vi "Read MP Registry Data.vi"(7 "Micropulse # In":i32, 8 "error in (no error)":errorcluster) -> (0 "error out":errorcluster, 2 "Micropulse Data":T2={"Instrument Type"=enum."MicroPulse 5", "Serial #"=0, "Sample Frequency"=enum."100MHz", "dt (us)"=0.0, "DOF"=enum."8-bit Mode", "Material Velocity"=1.0, "Asynch Reads"=enum."Disabled", "NUM of Tests"=0, "System Details"={"System Type"=enum."MicroPulse 5", "Serial No."=0, "Channels"={"Conv"=0, "PA"=0, "Extra"=0}, "Sample Frequency"={"Default"=0, "Actual"=0}, "Software Versions"="", "Data Output Format"={"Default"=enum."8-bit Mode", "Actual"=enum."8-bit Mode"}, "Temperatures"={"System"=0, "Processor"=0, "Slave Sys"=0, "Slave Proc"=0}, "Tx Buffer Size"=0, "System Error"="", "No. of Cards"=0, "DAC Gain"=0, "Uptimes"={"since Power"=0, "since RSTS"=0, "since SRST"=0}, "Voltages"=[], "Interface Cards"=[]}, "Gates"=[], "Encoders"=[], "CMD LUT"=variant, "Command List"=""} {"System Details"."Interface Cards"."FPGA - T" format="%.0f °C"; "System Details"."Interface Cards"."Board - T" format="%.0f °C"; "System Details"."Voltages"."Difference" format="%.2fV"; "System Details"."Voltages"."Measured" format="%.2fV"; "System Details"."Voltages"."Nominal" format="%.2fV"; "System Details"."DAC Gain" format="%.0fdB"; "System Details"."Tx Buffer Size" format="%.0fMB"; "System Details"."Temperatures"."Slave Proc" format="%.0f C"; "System Details"."Temperatures"."Slave Sys" format="%.0f C"; "System Details"."Temperatures"."Processor" format="%.0f C"; "System Details"."Temperatures"."System" format="%.0f C"; "System Details"."Sample Frequency"."Actual" format="%.0fMHz"; "System Details"."Sample Frequency"."Default" format="%.0fMHz"; "Encoders"."Encoder Filter" max=255; "Encoders"."Backlash Period (s)" min=0.0005 max=10.0 step=0.0005; "Encoders"."Multiplier" min=1 max=100000; "Encoders"."Counts/mm" min=1 max=100000; "Gates"."Insp Gates"."Max # Peaks" max=64000 step=100; "Gates"."Insp Gates"."Threshold" min=10 max=4095 step=10; "Gates"."Insp Gates"."Length (us)" min=0.0 max=96000.0 step=100.0; "Gates"."Insp Gates"."Start (us)" min=0.0 max=64000.0 step=100.0; "Gates"."Echo Gate"."Threshold" min=10 max=4095 step=10; "Gates"."Echo Gate"."Length (us)" min=0.0 max=96000.0 step=100.0; "Gates"."Echo Gate"."Start (us)" min=0.0 max=64000.0 step=100.0; "Gates"."Display Gate"."Length" min=0.0 max=64000.0 step=1000.0; "Gates"."Display Gate"."Start" min=0.0 max=64000.0 step=1000.0}, 3 "TCP config":T1={"Connection ID"=refnum, "IP address"="10.1.1.2", "host port"=1067, "OC timeout"=-1, "Read timeout"=0, "Write timeout"=0} {"Write timeout" format="%dms"; "Read timeout" format="%dms"; "OC timeout" format="%dms"}, 5 "Micropulse # Out":i32)   [LabVIEW 2026, in "MicroPulse_Driver.lvlib"]
doc: "The specified test(s) is repeated until a new mode (for example: STL or STX) is requested. The data is buffered for each cycle, i.e. if a single test is requested then data is output between each test, if all tests requested then data for each cycle of tests is buffered and output. The tests within a cycle are fired at the requested PRF (subject to gates set not being longer than the PRF). The next cycle will not start until this data has been output.\nParameters:\n<Tn> : Test number. An integer value from 0 to the maximum number of tests (default maximum is 1279 tests).\nTn = 0 for all conventional tests. If the S extension is used it applies to all tests in the sweep number specified: 1-32, 0 = all sweeps\n\nExample:\nNUM 100\nSTP 0 : MicroPulse sends data for tests 1 to 100 repeatedly\nSTL 1 : After completing the reporting of the data from the last test cycle, the MicroPulse enters STL mode on test 1."
uses:
  MicroPulse_Driver.lvlib
  Datatypes/MP-Registry Data-Cluster.ctl
  <instrlib>/MicroPulse/Public/Data/Datatypes/MP - instrument type.ctl
  Datatypes/MP - sample frequency.ctl
  Datatypes/MP - data output format.ctl
  Datatypes/MP - asynch read mode.ctl
  Datatypes/MP - general system status.ctl
  Datatypes/MP - interface card status.ctl
  Datatypes/subdatatypes/MP - Registry Gates.ctl
  Datatypes/MP - display gate.ctl
  Datatypes/MP - echo gate mode.ctl
  Datatypes/MP - echo gate parameters.ctl
  Datatypes/MP - multigate inspection gate parameters.ctl
  Datatypes/MP - hysteresis level.ctl
  Datatypes/MP - multigate mode.ctl
  Datatypes/MP - encoder settings.ctl
  Datatypes/MP - encoder type.ctl
  Datatypes/TCP config.ctl
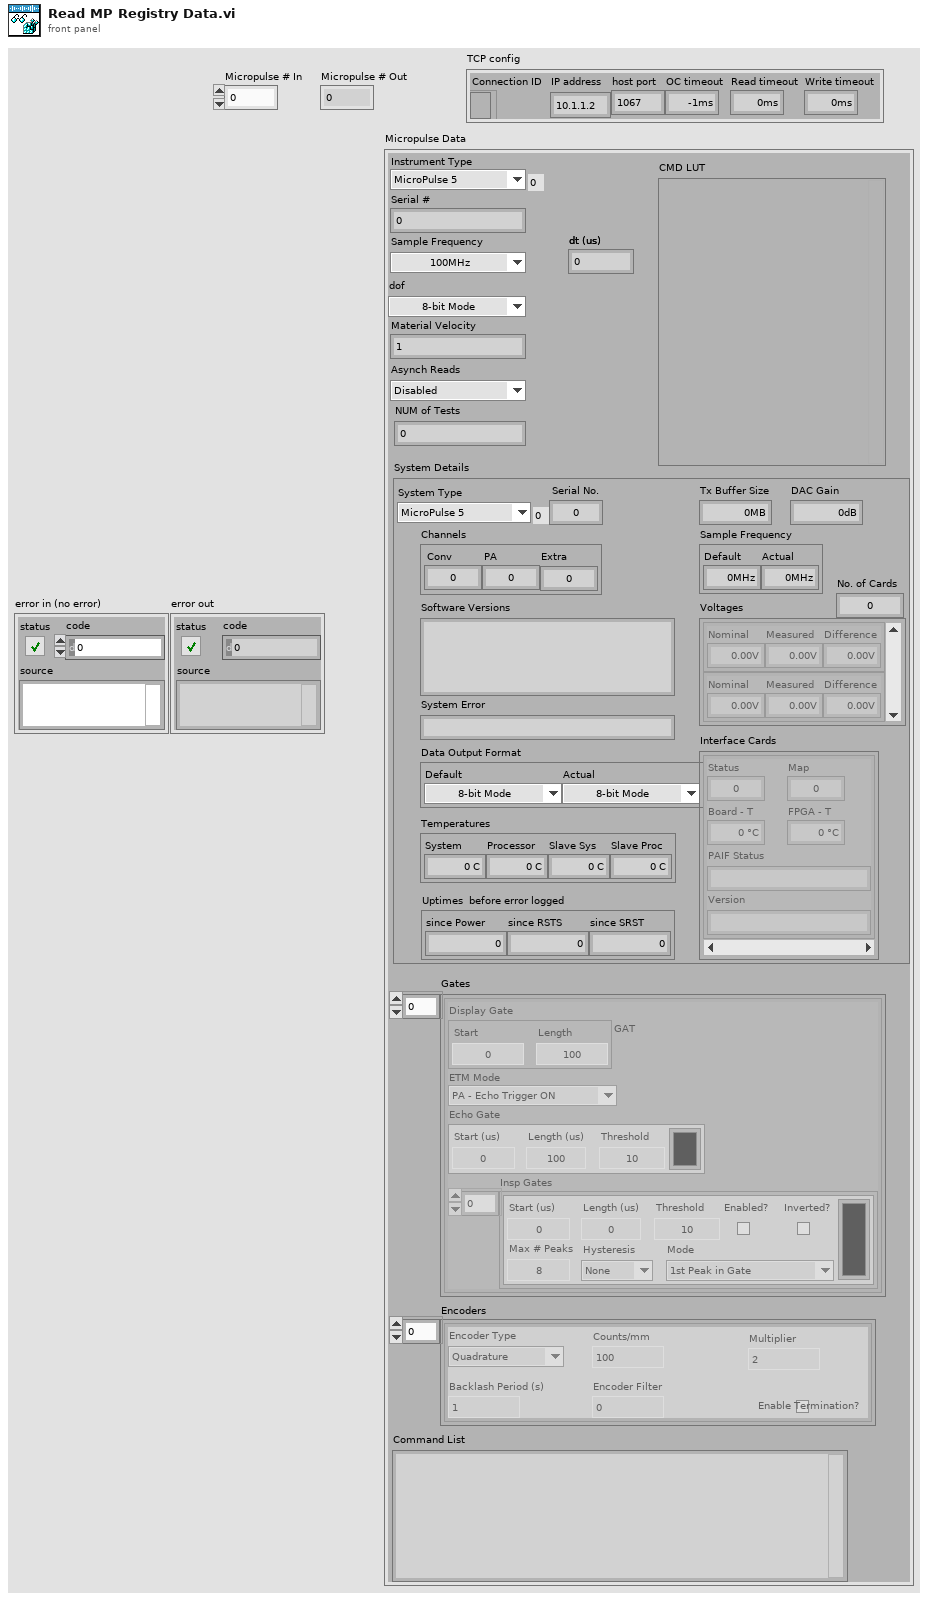
[diagram p1: front panel]
types:
  T1 = typedef "MicroPulse_Driver.lvlib/TCP config.ctl" = cluster{"Connection ID":refnum<k5>, "IP address":string, "host port":u16, "OC timeout":i32, "Read timeout":i32, "Write timeout":i32}
  T2 = typedef "MicroPulse_Driver.lvlib/MP-Registry Data-Cluster.ctl" = cluster{"Instrument Type":T3, "Serial #":u64, "Sample Frequency":T4, "dt (us)":dbl, "DOF":T5, "Material Velocity":dbl, "Asynch Reads":T6, "NUM of Tests":u32, "System Details":T7, "Gates":T9[], "Encoders":T16[], "CMD LUT":variant, "Command List":string}
  T3 = typedef "MicroPulse_Driver.lvlib/MP - instrument type.ctl" = enum16{"MicroPulse 5", "LT1", "LT2", "LTPA", "MPLT", "MicroPulse 6", "PipeScanner", "<MicroPulse>", "Micropulse 4", "Simulated Data"}
  T4 = typedef "MicroPulse_Driver.lvlib/MP - sample frequency.ctl" = enum16{"Use Default", "200MHz (LT2 only)", "100MHz", "50MHz", "25MHz", "10MHz"}
  T5 = typedef "MicroPulse_Driver.lvlib/MP - data output format.ctl" = enum16{"", "8-bit Mode", "10-bit Mode", "12-bit Mode", "16-bit Mode", "8-bit Log Mode", "12-bit Packed Mode"}
  T6 = typedef "MicroPulse_Driver.lvlib/MP - asynch read mode.ctl" = enum16{"Disabled", "Enabled"}
  T7 = typedef "MicroPulse_Driver.lvlib/MP - general system status.ctl" = cluster{"System Type":T3, "Serial No.":u64, "Channels":cluster{"Conv":u8, "PA":u16, "Extra":u32}, "Sample Frequency":cluster{"Default":u8, "Actual":u8}, "Software Versions":string, "Data Output Format":cluster{"Default":T5, "Actual":T5}, "Temperatures":cluster{"System":u8, "Processor":u8, "Slave Sys":u8, "Slave Proc":u8}, "Tx Buffer Size":u32, "System Error":string, "No. of Cards":u8, "DAC Gain":i16, "Uptimes":cluster{"since Power":u32, "since RSTS":u32, "since SRST":u32}, "Voltages":cluster{"Nominal":dbl, "Measured":dbl, "Difference":dbl}[], "Interface Cards":T8[]}
  T8 = typedef "MicroPulse_Driver.lvlib/MP - interface card status.ctl" = cluster{"Status":u8, "Map":u8, "Board - T":u8, "FPGA - T":u8, "PAIF Status":string, "Version":string}
  T9 = typedef "MicroPulse_Driver.lvlib/MP - Registry Gates.ctl" = cluster{"Display Gate":T10, "ETM Mode":T11, "Echo Gate":T12, "Insp Gates":T13[]}
  T10 = typedef "MicroPulse_Driver.lvlib/MP - display gate.ctl" = cluster{"Start":dbl, "Length":dbl}
  T11 = typedef "MicroPulse_Driver.lvlib/MP - echo gate mode.ctl" = enum16{"Echo Trigger OFF", "Echo Gate Display Mode", "Echo Trigger ON", "Multi Gate or FMC Mode", "Reserved", "PA - Echo Trigger ON"}
  T12 = typedef "MicroPulse_Driver.lvlib/MP - echo gate parameters.ctl" = cluster{"Start (us)":dbl, "Length (us)":dbl, "Threshold":u16, "Colour":u32}
  T13 = typedef "MicroPulse_Driver.lvlib/MP - multigate inspection gate parameters.ctl" = cluster{"Start (us)":dbl, "Length (us)":dbl, "Threshold":u16, "Enabled?":bool, "Max # Peaks":u16, "Hysteresis":T14, "Mode":T15, "Inverted?":bool, "Colour ":u32}
  T14 = typedef "MicroPulse_Driver.lvlib/MP - hysteresis level.ctl" = enum16{"None", "3dB", "6dB", "9dB", "12dB"}
  T15 = typedef "MicroPulse_Driver.lvlib/MP - multigate mode.ctl" = enum16{"1st Peak in Gate", "Largest Peak In Gate", "All Peaks In Gate", "1st Threshold Crossing"}
  T16 = typedef "MicroPulse_Driver.lvlib/MP - encoder settings.ctl" = cluster{"Encoder Type":T17, "Counts/mm":u32, "Enable Termination?":bool, "Multiplier":u32, "Backlash Period (s)":dbl, "Encoder Filter":u32}
  T17 = typedef "MicroPulse_Driver.lvlib/MP - encoder type.ctl" = enum16{"Quadrature", "Step/Direction"}
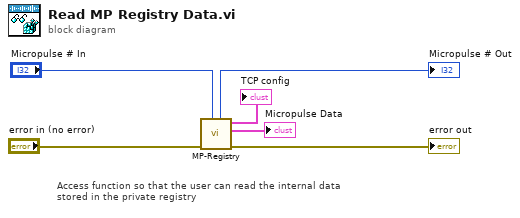
[diagram p0: block diagram]
diagram:
  # "Access function so that the user can read the internal data\nstored in the private registry"
  n1 = call "MP-Registry.vi"("Micropulse # In"="Micropulse # In", "error in (no error)"="error in (no error)") -> ("error out"=→"error out":errorcluster, "Micropulse Data"=→"Micropulse Data":T2, "TCP config"=→"TCP config":T1, "Micropulse # Out"=→"Micropulse # Out":i32)  [unwired: 6 in]
